vi "SysDef.Create.FromPrevious.vi"(8 "error in (no error)":errorcluster, 10 "Path in":path, 11 "Device Item Ref in":T1 format="%.0x") -> (0 "error out":errorcluster, 3 "Ref out":T1 format="%.0x")   [LabVIEW 2015, in "Diagnostics Addon System Explorer.lvlib"]
uses:
  Diagnostics Addon System Explorer.lvlib
  <vilib>/NI Veristand/Custom Device API/Custom Device Item Ref.ctl
  <vilib>/NI VeriStand/Custom Device API/Custom Device API.lvlib
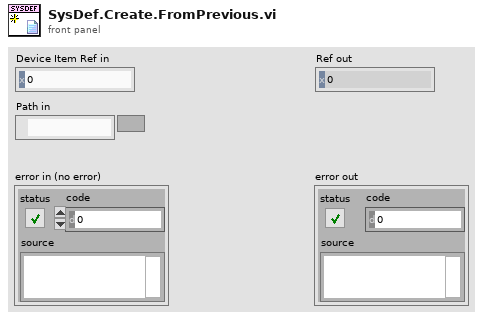
[diagram p1: front panel]
types:
  T1 = typedef "Custom Device API.lvlib/Custom Device Item Ref.ctl" = u64
  T2 = typedef "Diagnostics Addon System Explorer.lvlib/SysDef.Export.ctl" = cluster{"Name":string, "Description":string, "Diagnostics Basic Configuraiton":T3, "DID Outputs":T8, "DID Inputs":T8, "PID Outputs":T8, "PID Inputs":T8, "DPIDs":T11, "DTC":T15, "NI 986x Support":T19, "Commands":T20, "Status":T21, "IO Controls":T22, "Routines":T25, "Memory Outputs":T8, "Memory Inputs":T8, "User Defined":T27}
  T3 = typedef "Diagnostics Addon Shared.lvlib/CAN.ctl" = cluster{"Interface":T4, "Baud Rate":u32, "Diagnostic Protocol":T5, "Transport Protocol":T6, "Transmit ID":u32, "Receive ID":u32, "Transmit Extension":u8, "Receive Extension":u8, "Receive UUDT ID":u32, "Enable Stream":bool, "VW TP Channel ID":u32, "Fill Frame":bool, "Fill Byte":u8, "Termination":bool, "LIN Cluster":refnum<k21>, "NAD":u8, "IO Mode":u32, "Max DLC":u16, "FD Baud Rate":u32, "Security":T7}
  T4 = typedef "Diagnostics Addon Shared.lvlib/CAN.Interface.ctl" = string
  T5 = typedef "Diagnostics Addon Shared.lvlib/Protocol.ctl" = enum16{"GMLAN", "KWP-2000", "UDS", "User-Defined"}
  T6 = typedef "Diagnostics Addon Shared.lvlib/Transport.ctl" = enum16{"ISO TP - Normal Mode", "ISO TP - Mixed Mode", "VW TP 2.0", "Diagnostics on IP", "ISO TP LIN"}
  T7 = typedef "Diagnostics Addon Shared.lvlib/Security.ctl" = cluster{"Source DLL Path":path, "Security Level":u8, "Target DLL Path":path}
  T8 = typedef "Diagnostics Addon System Explorer.lvlib/Frames.Export.ctl" = cluster{"Description":string, "Frames":T9[]}
  T9 = typedef "Diagnostics Addon System Explorer.lvlib/Frame.Export.ctl" = cluster{"Name":string, "Description":string, "ID":u32, "Signals":T10[]}
  T10 = typedef "Diagnostics Addon Shared.lvlib/Signal.ctl" = cluster{"Start Bit":u32, "Length":u32, "Scaling Factor":dbl, "Scaling Offset":dbl, "Minimum":dbl, "Maximum":dbl, "Data Type":u32, "Byte Order":u32, "Default Value":dbl, "Name":string, "Units":string, "Description":string}
  T11 = typedef "Diagnostics Addon System Explorer.lvlib/DPIDs.Export.ctl" = cluster{"Description":string, "DPIDs":T12[]}
  T12 = typedef "Diagnostics Addon System Explorer.lvlib/DPID.Export.ctl" = cluster{"Name":string, "Description":string, "DPID":T13}
  T13 = typedef "Diagnostics Addon Shared.lvlib/DPID.ctl" = cluster{"DPID ID":u8, "Speed":T14, "PIDs":u16[]}
  T14 = typedef "Diagnostics Addon Shared.lvlib/DPID.Rate.ctl" = enum16{"Slow", "Medium", "Fast"}
  T15 = typedef "Diagnostics Addon System Explorer.lvlib/DTC.Export.ctl" = cluster{"Description":string, "Settings":T16, "DTC Control":T18, "Created DTCs":u32}
  T16 = typedef "Diagnostics Addon Shared.lvlib/DTC.Settings.ctl" = cluster{"Descriptor":T17, "Value.Code":dbl[], "Value.String":string[], "Status.Code":dbl[], "Status.String":string[]}
  T17 = typedef "Diagnostics Addon Shared.lvlib/DTC.Descriptor.ctl" = cluster{"DTC Byte Length":i32, "Status Byte Length":i32, "Add Data Byte Length":i32, "Byte Order":enum16{"Motorola", "Intel"}}
  T18 = typedef "Diagnostics Addon System Explorer.lvlib/DTCControl.Export.ctl" = cluster{"Description":string, "Signals":T10[]}
  T19 = typedef "Diagnostics Addon Shared.lvlib/986x.ctl" = cluster{"Enable":bool, "RIO Device":string, "Bitfile":path}
  T20 = typedef "Diagnostics Addon System Explorer.lvlib/Command.Export.ctl" = cluster{"Description":string}
  T21 = typedef "Diagnostics Addon System Explorer.lvlib/Status.Export.ctl" = cluster{"Description":string}
  T22 = typedef "Diagnostics Addon System Explorer.lvlib/IOControls.Export.ctl" = cluster{"Description":string, "IO Control Array":T23[]}
  T23 = typedef "Diagnostics Addon System Explorer.lvlib/IO.Export.ctl" = cluster{"Name":string, "Description":string, "ID":u16, "Signals":T24}
  T24 = typedef "Diagnostics Addon System Explorer.lvlib/CmdResp.Export.ctl" = cluster{"Cmd":T10[], "Response":T10[]}
  T25 = typedef "Diagnostics Addon System Explorer.lvlib/Routines.Export.ctl" = cluster{"Description":string, "Routine Array":T26[]}
  T26 = typedef "Diagnostics Addon System Explorer.lvlib/Routine.Export.ctl" = cluster{"Name":string, "Description":string, "ID":u16, "Start Parameters":T24, "Request Parameters":T24, "Stop Parameters":T24}
  T27 = typedef "Diagnostics Addon System Explorer.lvlib/UserDefined.Export.ctl" = cluster{"Description":string, "Groups":T28[]}
  T28 = typedef "Diagnostics Addon System Explorer.lvlib/UserDefined.Group.Export.ctl" = cluster{"Name":string, "Description":string, "Messages":T29[]}
  T29 = typedef "Diagnostics Addon System Explorer.lvlib/UserDefined.Group.Message.Export.ctl" = cluster{"Name":string, "Description":string, "Signals":T24}
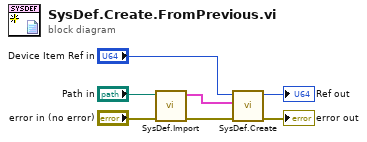
[diagram p0: block diagram]
diagram:
  n1 = call "SysDef.Import.vi"("error in (no error)"="error in (no error)", "Path in"="Path in") -> ("error out"=w5:errorcluster, "Configuration"=w1:T2)  [unwired: 8 in]
  n2 = call "SysDef.Create.vi"("error in (no error)"=w5, "Configuration"=w1, "Device Item Ref in"="Device Item Ref in") -> ("error out"=→"error out":errorcluster, "Device Item Ref out"=→"Ref out":T1)  [unwired: 7 in]
